vi "Exercicio 1.vi"() -> ()   [LabVIEW 2019]
panel:
  out "Temperatura":dbl
  in  "Resistência":dbl
  in  "stop":bool
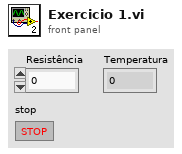
[diagram p1: front panel]
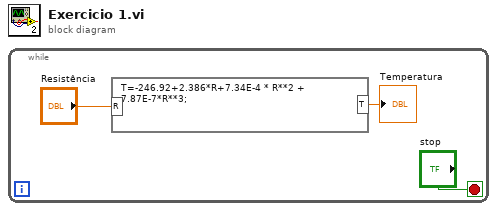
[diagram p0: block diagram]
diagram:
  n1 = while {
    stop <- "stop" stop-if-true
    n2 = formula code="T=-246.92+2.386*R+7.34E-4 * R**2 + 7.87E-7*R**3;"("R"="Resistência") -> ("T"=→"Temperatura":dbl)
  }
